vi "Dequeue Message.vi"(6 "Timeout (-1)":i32, 8 "error in (no error)":errorcluster, 11 "Message Queue in":refnum<class "Message Queue.lvclass">) -> (0 "error out":errorcluster, 1 "Data":variant, 2 "Msg":string, 3 "Message Queue out":refnum<class "Message Queue.lvclass">, 4 "Timed Out?":bool)   [LabVIEW 2019, in "Network Interface.lvlib" / "Message Queue.lvclass"]
uses:
  <vilib>/gpm_packages/@cs/Network-Sink/Source/Network Interface/Message Queue/Message Queue.lvclass
  <vilib>/gpm_packages/@cs/Network-Sink/Source/Network Interface/Message Queue/Message Queue.lvclass/Message Queue.ctl
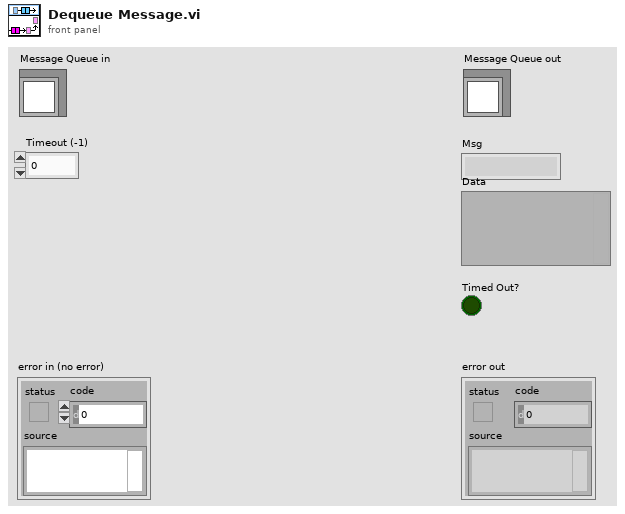
[diagram p1: front panel]
types:
  T1 = typedef "Network Sink.lvlib/Message Cluster.ctl" = cluster{"Msg":string, "Data":variant}
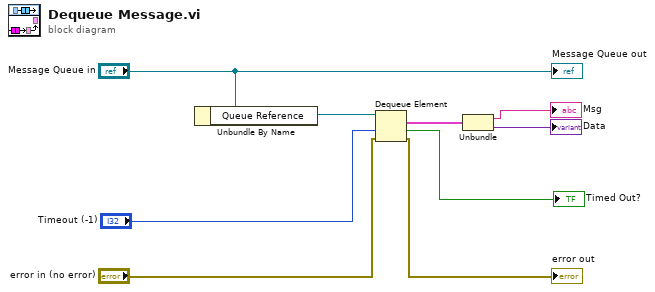
[diagram p0: block diagram]
diagram:
  n1 = Unbundle By Name("Message Queue in") -> ("Queue Reference"=w8:refnum<queue>)
  n2 = Dequeue Element(queue=w8, timeout in ms (-1)="Timeout (-1)", error in (no error)="error in (no error)") -> (element=w5:T1, timed out?=→"Timed Out?":bool, error out=→"error out":errorcluster)  [unwired: 1 out]
  n3 = Unbundle(w5) -> ("Msg"=→"Msg":string, "Data"=→"Data":variant)
  "Message Queue out" <- "Message Queue in"
